vi "LoadFileFromMIDAS.vi"(9 "Filename":string, 10 "Project Name":string, 11 "File":path) -> (1 "MD5 is same":bool, 2 "data":string)   [LabVIEW 2018, in "feGEM DataPacker.lvlib"]
uses:
  feGEM DataPacker.lvlib
  14431f1c-0a81-40c8-aa13-bea41e9e81ac.vi
  14431f1c-0a81-40c8-aa13-bea41e9e81ac.vi/1fbeea10-0a75-4c84-8769-58e1ad49c331.vi
panel:
  out "length":i32
  out "error out":errorcluster
  in  "MD5 (optional)":string
  out "size (in bytes) in memory":i32
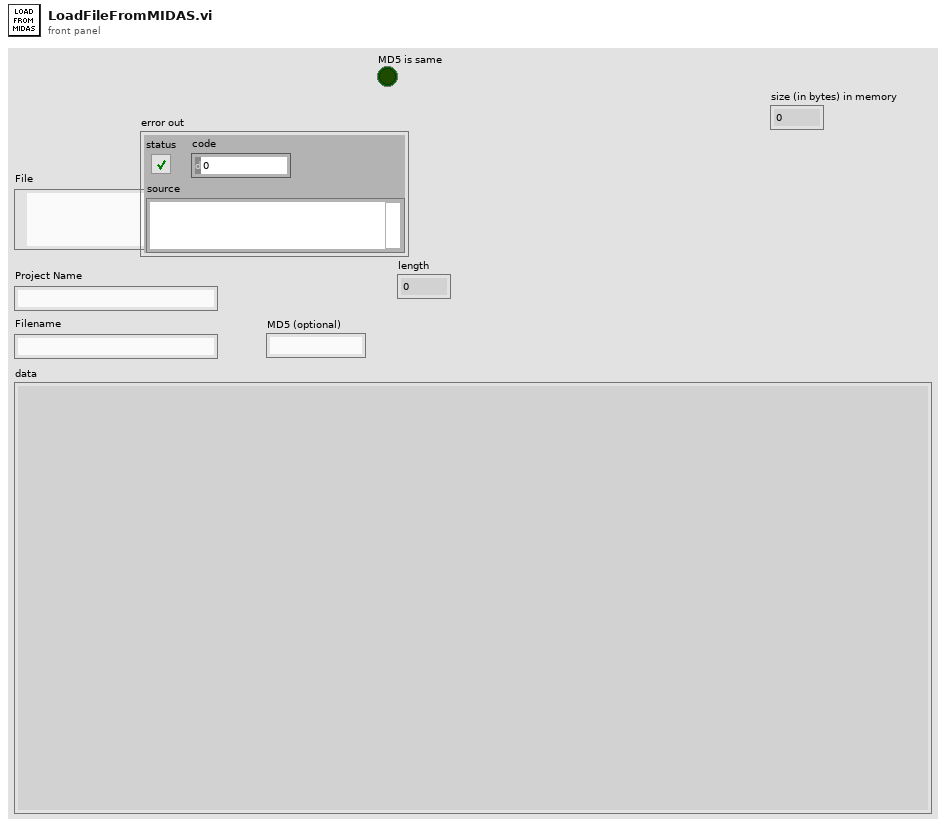
[diagram p1: front panel]
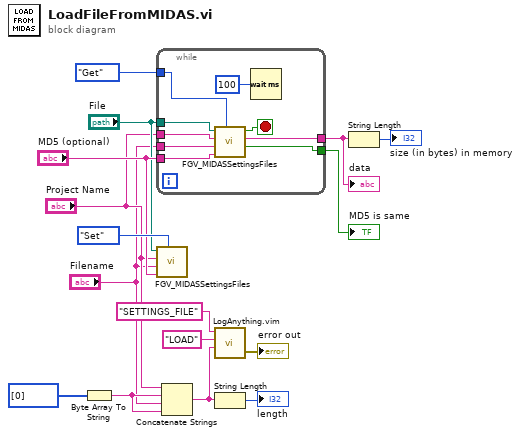
[diagram p0: block diagram]
diagram:
  n1 = Byte Array To String(unsigned byte array=u8[] [0]) -> (string=w8:string)
  n2 = while {
    tunnel: "Filename" -> [w24]
    tunnel: "MD5 (optional)" -> [w23]
    tunnel: "File" -> [w22]
    tunnel: enum16{"AddData", "Set", "Get"}."Get" ("Enum") -> [w21]
    tunnel: [w19] -> w11
    tunnel: "Project Name" -> [w25]
    tunnel: [w20] -> w10
    stop <- w18 stop-if-true
    n3 = call "FGV_MIDASSettingsFiles.vi"("Enum"=w21, "MD5 (optional)"=w23, "FileName"=w24, "ProjectName"=w25, "Path"=w22) -> ("MD5 is same"=w19:bool, "BinaryData"=w20:string, "HaveData"=w18:bool)  [unwired: 4 in]
    n4 = Wait (ms)(milliseconds to wait=u32 100) -> ()  [unwired: 1 out]
  }
  "data" <- w10
  "MD5 is same" <- w11
  n5 = call "FGV_MIDASSettingsFiles.vi"("Enum"=enum16{"AddData", "Set", "Get"}."Set", "MD5 (optional)"="MD5 (optional)", "FileName"="Filename", "ProjectName"="Project Name", "Path"="File") -> ()  [unwired: 4 in, 3 out]
  n6 = Concatenate Strings("Project Name", w8, "Filename", w8) -> (w3:string)
  n7 = call "LogAnything.vim"("Array"=w3, "Var Name"="LOAD", "Category"="SETTINGS_FILE") -> ("error out"=→"error out":errorcluster)  [unwired: 4 in]
  n8 = String Length(string=w3) -> (length=→"length":i32)
  n9 = String Length(string=w10) -> (length=→"size (in bytes) in memory":i32)
